vi "GA Cmp Pluse.vi"(6 "nTime2":i16, 7 "nTime1":i16, 8 "error in (no error)":errorcluster caption="错误输入（无错误）", 9 "nPluseType2":i16, 10 "nPluseType1":i16, 11 "nChannel":i16) -> (0 "error out":errorcluster caption="错误输出", 3 "function return":i32)   [LabVIEW 2015, in "GAS.lvlib"]
doc: "extern \"C\" __declspec(dllimport) int GA_CmpPluse(short nChannel, short nPluseType1, short nPluseType2, short nTime1,short nTime2);"
uses:
  <userlib>/BP_GAS/GAS.lvlib
  <userlib>/BP_GAS/GAS.dll
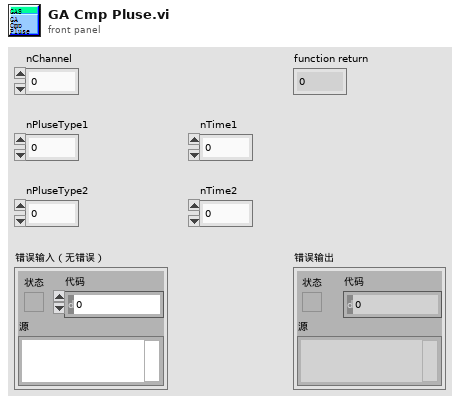
[diagram p1: front panel]
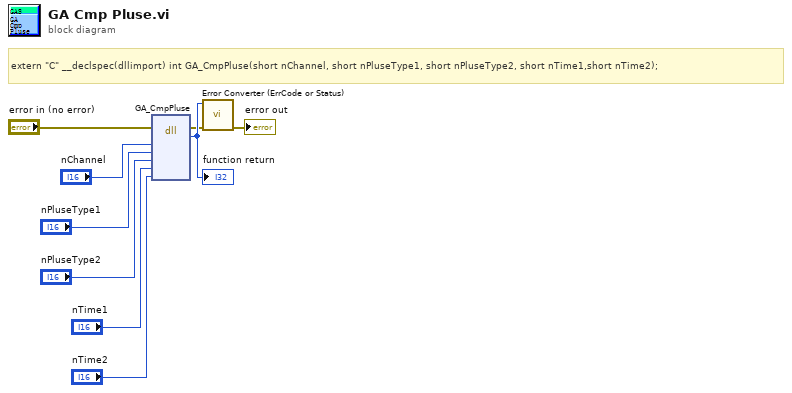
[diagram p0: block diagram]
diagram:
  # "extern \"C\" __declspec(dllimport) int GA_CmpPluse(short nChannel, short nPluseType1, short nPluseType2, short nTime1,short nTime2);"
  n1 = dll-call lib="E:/Program Files (x86)/National Instruments/LabVIEW 2015/user.lib/BP_GAS/GAS.*" fn="GA_CmpPluse"(error in="error in (no error)", "nChannel"="nChannel", "nPluseType1"="nPluseType1", "nPluseType2"="nPluseType2", "nTime1"="nTime1", "nTime2"="nTime2") -> (error out=w2:errorcluster, w9:i32)  [unwired: 7 in, 1 out]
  "function return" <- w9
  n2 = call "Error Converter (ErrCode or Status).vi"("error in (no error)"=w2, "error code"=w9) -> ("error out"=→"error out":errorcluster)  [unwired: 9 in]
